vi "Dashboard Main.vi"() -> ()   [LabVIEW 2019]
uses:
  <vilib>/Utility/miscctls.llb/LVRowAndColumnTypeDef.ctl
  <vilib>/event_ctls.llb/eventvkey.ctl
  <vilib>/Rock Robotics/Network Tables/NT Read Numeric Array.vi
  <vilib>/Rock Robotics/WPI/Dashboard/WPI_DashboardLogging Global.vi
  <vilib>/Rock Robotics/Network Tables/NT Read Variant.vi
panel:
  out "NT Connection":bool
  in  "Camera Settings Right":T1={"Frame Rate"=30, "Compression"=30, "Size"=1, "DB Camera Config"=FALSE} {"Frame Rate" scale=1.0..30.0; "Compression" scale=100.0..-1.0; "Size" items=["640x480", "320x240", "160x120"]}
  in  "Camera Name Right":string(combo)="No Camera Selection"
  out "Camera Perf":string
  in  "Camera Settings":T1={"Frame Rate"=30, "Compression"=30, "Size"=1, "DB Camera Config"=FALSE} {"Frame Rate" scale=1.0..30.0; "Compression" scale=100.0..-1.0; "Size" items=["640x480", "320x240", "160x120"]}
  in  "TCP":refnum<k5>
  in  "Rec Mode":enum32{"Stop", "Record", "Playback"}(radio)
  out "Robot IP":string
  out "Image Message":string="Timeout in Camera Communications"
  in  "Dashboard Tab":T2(tab)
  out "SensorData":T3={"LeftDistance"=3962.033502451172, "RightDistance"=3821.920006201172, "LeftVelocity"=0.0, "RightVelocity"=0.0, "Angle"=-59.4, "Location"={597.0445781606653, 278.6835922961287}}
  out "Mode":T4(ring)=enum."Auto Disabled"
  out "Right Camera Perf":cluster{"Bandwidth (Mbps)":dbl, "FPS":dbl}
  out "AutoFilesOnRobot":string[](array[string])
  in  "WaitAtStartOfAuto":dbl
  in  "AutoFileName (No .txt)":string
  out "Camera Image Right":T5(plugin-control)
  in  "DB/String 9":string
  in  "DB/String 8":string
  in  "DB/String 7":string
  in  "DB/String 6":string
  in  "DB/String 5":string
  in  "DB/String 4":string
  in  "DB/String 3":string
  in  "DB/String 2":string
  in  "DB/String 1":string
  in  "DB/String 0":string
  in  "DB/Slider 0":dbl(slide) scale=0.0..5.0
  in  "DB/Slider 1":dbl(slide) scale=0.0..5.0
  in  "DB/Slider 2":dbl(slide) scale=0.0..5.0
  in  "DB/Slider 3":dbl(slide) scale=0.0..5.0
  out "DB/LED 3":bool
  out "DB/LED 2":bool
  out "DB/LED 1":bool
  out "DB/LED 0":bool
  in  "DB/Button 3":bool
  in  "DB/Button 2":bool
  in  "DB/Button 1":bool
  in  "DB/Button 0":bool caption="New Name"
  in  "Test Slider":dbl(slide) scale=0.0..100.0 scale format="%#_3g"
  in  "On/Off":bool caption="Solenoid"
  in  "Test Name":u16(ring) items=["Select the test to run..."]
  in  "Test Tree":string(tree)
  in  "Motor":cluster{"Value":dbl, "Enable":bool} {"Value" scale=-1.0..1.0 scale format="%#_3g"}
  out "Progress":T6 {"Test Progress" scale=0.0..100.0}
  in  "Rev/Fwd":cluster{"Forward":bool, "Reverse":bool}
  in  "Test Ring":u16(ring) items=["Monochrome", "Color"]
  out "Cmd Status":string
  in  "Execute Command":bool
  in  "Command Params":string[][](table)
  in  "Command Selection":i32(listbox)
  in  "CheckList":i32(listbox)
  out "Tree":string(tree)
  out "Camera Image":T5(plugin-control)
  in  "Camera Name":string(combo)="No Camera Selection"
  # "HW"
  # "HW"
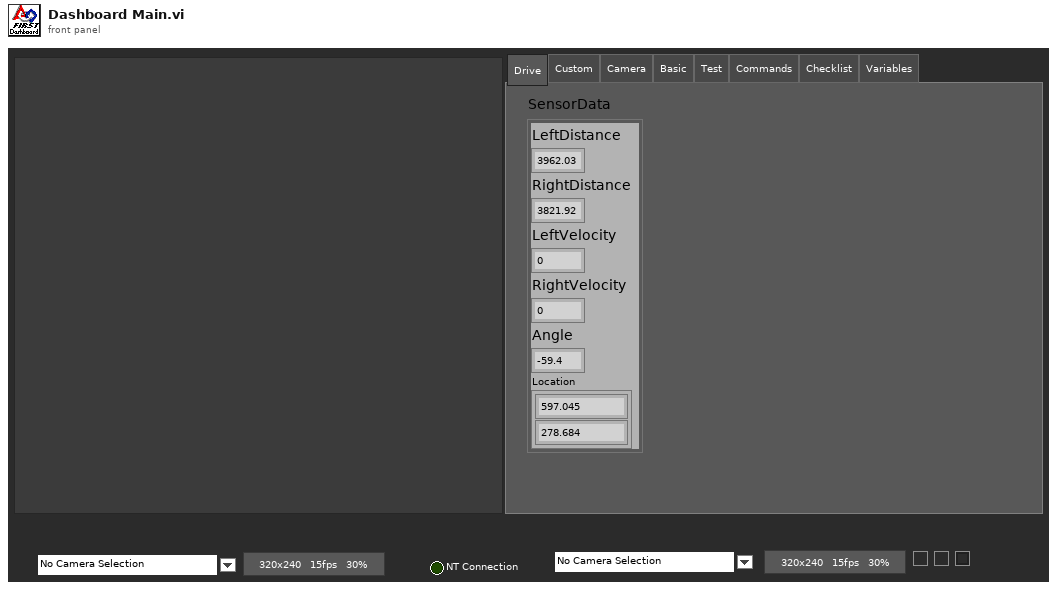
[diagram p1: front panel]
types:
  T1 = cluster{"Frame Rate":i32, "Compression":i32, "Size":u16, "DB Camera Config":bool}
  T2 = enum32{"Drive", "Custom", "Camera", "Basic", "Test", "Commands", "Checklist", "Variables"}
  T3 = cluster{"LeftDistance":dbl, "RightDistance":dbl, "LeftVelocity":dbl, "RightVelocity":dbl, "Angle":dbl, "Location":cluster{dbl, dbl}}
  T4 = enum8{"Tele-Op Disabled", "Tele-Op Enabled", "Auto Disabled", "Auto Enabled", "Test Disabled", "Test Enabled", "Disconnected", "No Code", "E-Stop"}
  T5 = typedef "IMAQ Image.ctl" = refnum<image>
  T6 = cluster{"Test Progress":u8, "Test Progress Text":string}
  T7 = cluster{"Save Path":path, "Interval (s)":dbl, "Keep":i32}
  T8 = typedef "Image Type" = u32
  T9 = cluster{"IDs":cluster{"RPC field ID":u16, "Unique ID":u16}, "String":string}
  T10 = cluster{"Camera Image":refnum<vi>, "Dashboard Tab":refnum<vi>, void, "Rec Mode":refnum<vi>, "Test Slider":refnum<vi>, "On/Off ":refnum<vi>, "Test Ring":refnum<vi>, "Rev/Fwd":refnum<vi>, "Test Name":refnum<vi>, "Motor":refnum<vi>, "Progress":refnum<vi>, "CheckList":refnum<vi>, "Tree":refnum<vi>, "Test Tree":refnum<vi>, "Command Params":refnum<vi>, "Command Selection":refnum<vi>, "Execute Command":refnum<vi>, "Cmd Status":refnum<vi>, "Camera Settings":refnum<vi>, "Camera Name":refnum<vi>, "Camera Perf":refnum<vi>, "Camera Settings Right":refnum<vi>, "Camera Name Right":refnum<vi>, "Camera Image Right":refnum<vi>}
  T11 = cluster{"Error Strings":string, "Disable Counts":cluster{u16, u16}, "Rail Faults":cluster{u16, u16, u16}, "Robot IP":string, "DB Mode":u8, "Event Info":cluster{"Name":string, "Type":u8, "Number":u16, "Replay":u8}}
  T12 = cluster{"Storage":cluster{"Disk Free":u64, "RAM Block":u32, "RAM free":u32}, "CPU Utilization":cluster{"CPU % ISR":sgl, "CPU % Time Crit":sgl, "CPU % Timed Str":sgl, "CPU % High":sgl, "CPU % Above":sgl, "CPU % Normal":sgl, "CPU % Low":sgl}, "CAN":cluster{"% Bus Utilization":sgl, "Bus Off Cnt":u32, "TX_FIFO Full Cnt":u32, "Receive Error Cnt":u8, "Transmit Error Cnt":u8}, "HID":cluster{"HID Outputs":u32, "Rumble Low":u16, "Rumble High":u16}[]}
  T13 = cluster{"Status bits":cluster{"Test Mode":bool, "Autonomous":bool, "Enabled":bool, "Code Start":bool, "Brownout":bool, "Reserved 2":bool, "Reserved 3":bool, "E-Stop":bool}, "Code Trace":cluster{"Disabled":bool, "TeleOp":bool, "Auto":bool, "Test":bool}, "Controller Type":enum16{"unknown", "cRIO", "roboRio"}, "Code?":enum16{"unknown", "noCode", "code"}, "Battery V":dbl}
  T14 = cluster{"Control Bits":cluster{"TestMode":bool, "Autonomous":bool, "Enabled":bool, "FMS Present":bool, bool, bool, bool, "E-Stop":bool}, "Team Station ":u8, "Countdown":sgl, "Joystick Values":cluster{"Axes":dbl[], "Buttons":bool[], "POVs":i16[]}[]}
  T15 = cluster{"Axes":dbl[], "Buttons":bool[], "POVs":i16[]}[]
  T16 = cluster{"Axes":dbl[], "Buttons":bool[], "POVs":i16[]}
  T17 = cluster{"Global Rectangle":i32[], "Contours":cluster{"Contour Type":u32, "ROI Type":u32, "Points":i32[]}[]}
  T18 = cluster{"Camera Name":string, string, "Saved DB Images Info":cluster{"Save Path":path, "Interval (s)":dbl, "Keep":i32}}
  T19 = cluster{"Camera Name Right":string, string, "Saved DB Images Info":cluster{"Save Path":path, "Interval (s)":dbl, "Keep":i32}}
  T20 = cluster{"Operation":enum16{"Update", "Clear"}, "Color Box":u32}[]
  T21 = typedef "eventvkey.ctl" = enum16{"ASCII", "Enter", "Return", "Shift", "Ctrl", "Alt", "Cmd", "Opt", "Caps", "NumLock", "Clear", "Break", "Up", "Down", "Left", "Right", "Insert", "Delete", "Home", "End", "PageUp", "PageDown", "Escape", "Help", "Pause", "ScrollLock", "F1", "F2", "F3", "F4", "F5", "F6", "F7", "F8", "F9", "F10", "F11", "F12", "F13", "F14", "F15", "F16", "F17", "F18", "F19", "F20", "F21", "F22", "F23", "F24", "Play", "VolumeUp", "VolumeDown", "Mute", "Two Byte Char"}
  T22 = cluster{"Image Size":bool, "Image Type":bool, "Pixel Value":bool, "ROI Information":bool, "Zoom Factor":bool}
  T23 = cluster{"Operation":enum16{"Update", "Clear"}, "Color Box":u32}
  T24 = typedef "LVRowAndColumnTypeDef.ctl" = cluster{"Row":i32, "Column":i32}
  T25 = cluster{"Shift":bool, "Ctrl":bool, "Alt":bool, "Cmd":bool, "Opt":bool}
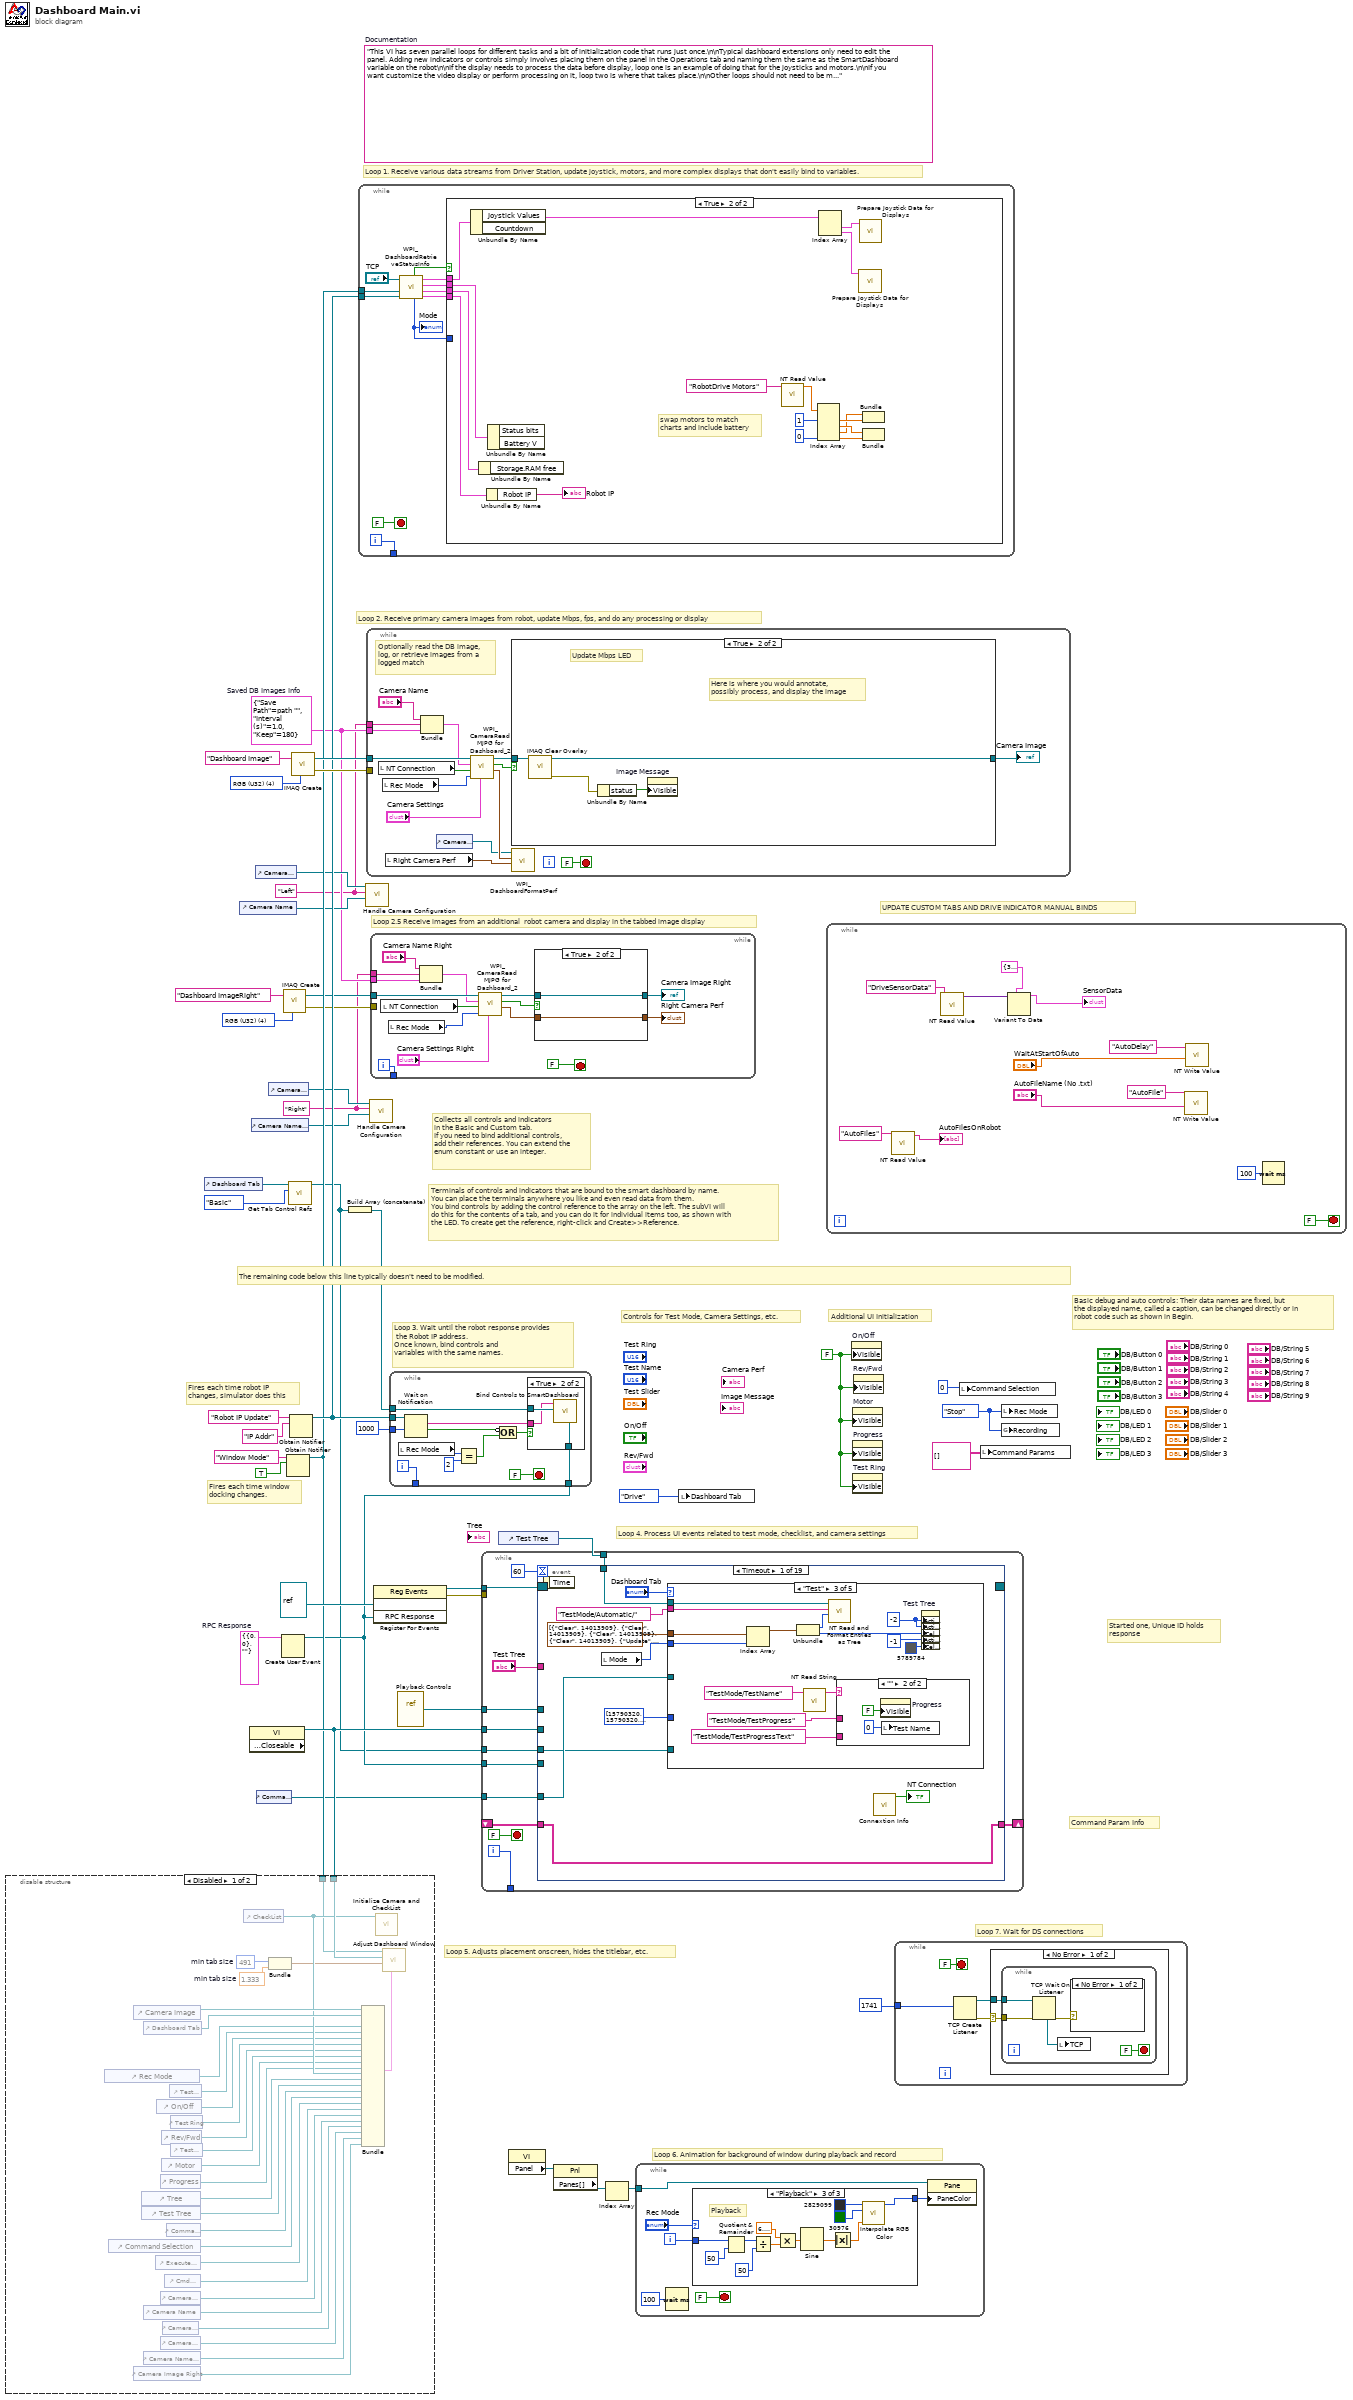
[diagram p0: block diagram]
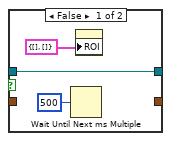
[diagram p3: hidden frame]
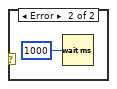
[diagram p4: hidden frame]
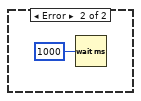
[diagram p5: hidden frame]
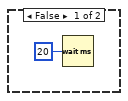
[diagram p6: hidden frame]
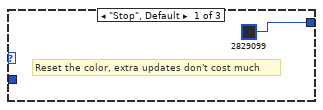
[diagram p7: hidden frame]
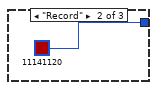
[diagram p8: hidden frame]
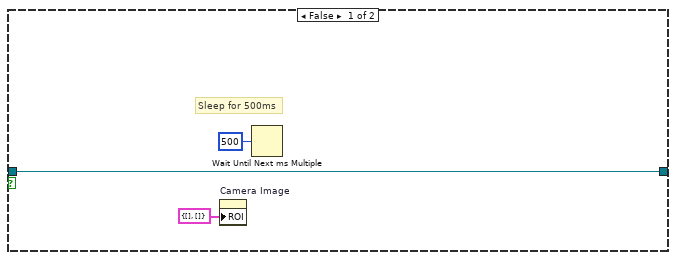
[diagram p10: hidden frame]
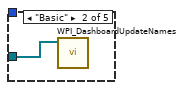
[diagram p12: hidden frame]
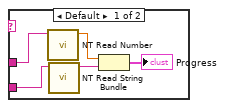
[diagram p13: hidden frame]
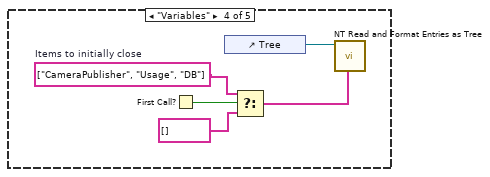
[diagram p14: hidden frame]
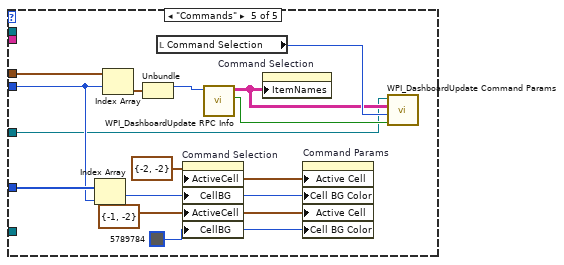
[diagram p15: hidden frame]
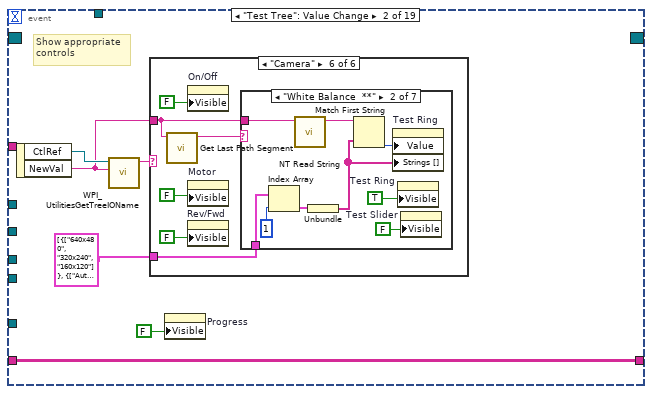
[diagram p16: hidden frame]
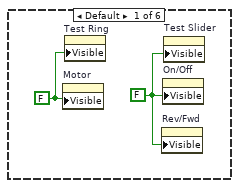
[diagram p17: hidden frame]
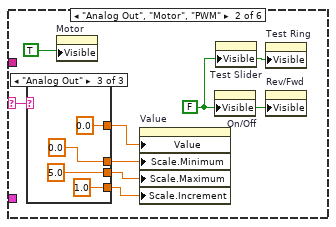
[diagram p18: hidden frame]
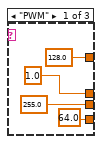
[diagram p19: hidden frame]
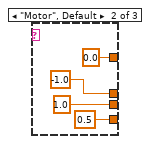
[diagram p20: hidden frame]
diagram:
  w4 = T7 {"Save Path"=path "", "Interval (s)"=1.0, "Keep"=180}  # Saved DB Images Info
  w3 = "Right"
  w2 = "Left"
  w9 = T8 4 items=["Grayscale (U8)", "Grayscale (I16)", "Grayscale (SGL)", "Complex (CSG)", "RGB (U32)", "HSL (U32)", "RGB (U64)"] ("Image Type")
  w18 = T9 {"IDs"={"RPC field ID"=0, "Unique ID"=0}, "String"=""}  # RPC Response
  w27 = enum32{"Stop", "Record", "Playback"}."Stop" ("Rec Mode")
  w23 = FALSE ("Visible")
  (unwired) "This VI has seven parallel loops for different tasks and a bit of initialization code that runs just once.\n\nTypical dashboard extensions only need to edit the panel. Adding new indicators or controls simply involves placing them on the panel in the Operations tab and naming them the same as the SmartDashboard variable on the robot\n\nIf the display needs to process the data before display, loop one is an example of doing that for the joysticks and motors.\n\nIf you want customize the video display or perform processing on it, loop two is where that takes place.\n\nOther loops should not need to be modified. They are pretty standard, and document the task they perform."  # Documentation
  w44 = T8 4 items=["Grayscale (U8)", "Grayscale (I16)", "Grayscale (SGL)", "Complex (CSG)", "RGB (U32)", "HSL (U32)", "RGB (U64)"] ("Image Type")
  # "UPDATE CUSTOM TABS AND DRIVE INDICATOR MANUAL BINDS"
  # "Loop 2.5 Receive images from an additional  robot camera and display in the tabbed image display"
  # "Command Param Info"
  # "Started one, Unique ID holds\nresponse"
  # "Loop 7. Wait for DS connections"
  # "Basic debug and auto controls: Their data names are fixed, but\nthe displayed name, called a caption, can be changed directly or in\nrobot code such as shown in Begin."
  # "Controls for Test Mode, Camera Settings, etc."
  # "Additional UI Initialization"
  # "Loop 6. Animation for background of window during playback and record"
  # "Fires each time robot IP\nchanges, simulator does this"
  # "Fires each time window\ndocking changes."
  # "Collects all controls and indicators\nin the Basic and Custom tab.\nIf you need to bind additional controls,\nadd their references. You can extend the\nenum constant or use an integer."
  # "The remaining code below this line typically doesn't need to be modified."
  # "Loop 4. Process UI events related to test mode, checklist, and camera settings"
  # "Terminals of controls and indicators that are bound to the smart dashboard by name.\nYou can place the terminals anywhere you like and even read data from them.\nYou bind controls by adding the control reference to the array on the left. The subVI will\ndo this for the contents of a tab, and you can do it for individual items too, as shown with\nthe LED. To create get the reference, right-click and Create>>Reference."
  # "Loop 3. Wait until the robot response provides\n the Robot IP address.\nOnce known, bind controls and\nvariables with the same names."
  # "Loop 5. Adjusts placement onscreen, hides the titlebar, etc."
  # "Loop 1. Receive various data streams from Driver Station, update joystick, motors, and more complex displays that don't easily bind to variables."
  # "Loop 2. Receive primary camera images from robot, update Mbps, fps, and do any processing or display"
  n1 = control-ref of="Dashboard Tab"() -> (w25:refnum<vi>)
  n2 = control-ref of="Camera Name"() -> (w12:refnum<vi>)
  n3 = property class="VI" props=["Front Panel.Closeable"]() -> (reference out=w26:refnum<vi>)  [unwired: 2 in, 2 out]
  n4 = control-ref of="Camera Name Right"() -> (w5:refnum<vi>)
  n5 = control-ref of="Camera Settings"() -> (w13:refnum<vi>)
  n6 = control-ref of="Command Params"() -> (w14:refnum<vi>)
  n7 = control-ref of="Camera Settings Right"() -> (w6:refnum<vi>)
  n8 = Create User Event(user event datatype=w18) -> (user event=w15:refnum<user-event>)  [unwired: 1 in, 1 out]
  n9 = call "IMAQ Create"("Image Name"="Dashboard ImageRight", "Image Type"=w9) -> ("New Image"=w8:T5, "error out"=w7:errorcluster)  [unwired: 2 in, 1 out]
  n10 = Obtain Notifier(name (unnamed)="Window Mode", notification data type=TRUE) -> (notifier out=w21:refnum<notifier>)  [unwired: 2 in, 2 out]
  n11 = disable-structure shown="Disabled" {
    disable-tunnel: w26 -> [w73 _]
    disable-tunnel: w21 -> [w58 _]
    frame Disabled {
      w47 = 491  # min tab size
      w46 = 1.333  # min tab size
      n12 = control-ref of="Rec Mode"() -> (w64:refnum<vi>)
      n13 = control-ref of="Command Selection"() -> (w55:refnum<vi>)
      n14 = control-ref of="Camera Image Right"() -> (w48:refnum<vi>)
      n15 = control-ref of="Camera Image"() -> (w72:refnum<vi>)
      n16 = control-ref of="Tree"() -> (w68:refnum<vi>)
      n17 = control-ref of="Test Tree"() -> (w67:refnum<vi>)
      n18 = control-ref of="Dashboard Tab"() -> (w71:refnum<vi>)
      n19 = control-ref of="Camera Name"() -> (w52:refnum<vi>)
      n20 = control-ref of="Camera Name Right"() -> (w49:refnum<vi>)
      n21 = control-ref of="Execute Command"() -> (w56:refnum<vi>)
      n22 = control-ref of="On/Off"() -> (w62:refnum<vi>)
      n23 = control-ref of="Progress"() -> (w59:refnum<vi>)
      n24 = control-ref of="Camera Settings"() -> (w53:refnum<vi>)
      n25 = control-ref of="Camera Settings Right"() -> (w50:refnum<vi>)
      n26 = control-ref of="Rev/Fwd"() -> (w60:refnum<vi>)
      n27 = control-ref of="Motor"() -> (w65:refnum<vi>)
      n28 = control-ref of="Camera Perf"() -> (w51:refnum<vi>)
      n29 = control-ref of="Cmd Status"() -> (w54:refnum<vi>)
      n30 = control-ref of="Command Params"() -> (w57:refnum<vi>)
      n31 = control-ref of="Test Slider"() -> (w63:refnum<vi>)
      n32 = control-ref of="Test Ring"() -> (w61:refnum<vi>)
      n33 = control-ref of="Test Name"() -> (w66:refnum<vi>)
      n34 = control-ref of="CheckList"() -> (w69:refnum<vi>)
      n35 = Bundle("min tab size"=w47, "min tab size"=w46) -> (w45:cluster{"min tab size":i32, "min tab size":dbl})  [unwired: 1 in]
      n36 = Bundle("Camera Image"=w72, "Dashboard Tab"=w71, "Rec Mode"=w64, "Test Slider"=w63, "On/Off"=w62, "Test Ring"=w61, "Rev/Fwd"=w60, "Test Name"=w66, "Motor"=w65, "Progress"=w59, "CheckList"=w69, "Tree"=w68, "Test Tree"=w67, "Command Params"=w57, "Command Selection"=w55, "Execute Command"=w56, "Cmd Status"=w54, "Camera Settings"=w53, "Camera Name"=w52, "Camera Perf"=w51, "Camera Settings Right"=w50, "Camera Name Right"=w49, "Camera Image Right"=w48) -> (w70:T10)  [unwired: 2 in]
      n37 = call "Initialize Camera and CheckList.vi"("ListBox in"=w69) -> ()  [unwired: 11 in]
      n38 = call "Adjust Dashboard Window.vi"("Sizing Refnums"=w70, "Size Constraints"=w45, "VI"=w73, "WIn Mode"=w58) -> ()  [unwired: 8 in]
    }
    frame Enabled {
    }
  }
  n39 = call <vilib>:"Get Tab Control Refs.vi"("Page Index"=T2."Basic" ("Dashboard Tab"), "TabControl in"=w25) -> ("ControlsOnPage"=w11:refnum<vi>[])  [unwired: 9 in]
  n40 = Obtain Notifier(name (unnamed)="Robot IP Update", notification data type="IP Addr" ("name (unnamed)")) -> (notifier out=w22:refnum<notifier>)  [unwired: 2 in, 2 out]
  n41 = call "IMAQ Create"("Image Name"="Dashboard Image", "Image Type"=w44) -> ("New Image"=w42:T5, "error out"=w41:errorcluster)  [unwired: 2 in, 1 out]
  n42 = Build Array (concatenate)(w11) -> (w24:refnum<vi>[])
  n43 = while {
    tunnel: [w83] -> _
    tunnel: w22 -> [w77]
    tunnel: w21 -> [w74]
    i -> [w83]
    stop <- FALSE stop-if-true
    n44 = call <vilib>:"WPI_DashboardRetrieveStatusInfo.vi"("Binding Refnum"=w77, "Window Mode Notifier"=w74, "TCP Cnx"="TCP") -> ("Power and Errors"=w78:T11, "Robot Metrics"=w81:T12, "Status Info"=w82:T13, "Control Info"=w79:T14, "Robot Mode"=w76:T4, "Process?"=w80:bool)  [unwired: 3 in]
    "Mode" <- w76
    n45 = case shown="True" w80 {
      tunnel: w82 -> [_ w101]
      tunnel: w81 -> [_ w100]
      tunnel: w79 -> [_ w99]
      tunnel: w78 -> [_ w98]
      tunnel: w76 -> [_ _]
      frame False {
        n46 = Wait (ms)(milliseconds to wait=u32 20) -> ()  [unwired: 1 out]
      }
      frame True {
        # "swap motors to match\ncharts and include battery"
        n47 = Unbundle By Name(w99) -> ("Joystick Values"=w91:T15)  [unwired: 1 out]
        n48 = Unbundle By Name(w100) -> ()  [unwired: 1 out]
        n49 = Unbundle By Name(w98) -> ("Robot IP"=→"Robot IP":string)
        n50 = Unbundle By Name(w101) -> ()  [unwired: 2 out]
        n51 = call-poly <vilib>:"NT Read Value.vi"("Name"="RobotDrive Motors") -> ("Numeric Array"=w87:dbl[])  [unwired: 9 in, 1 out]
        n52 = Index Array(array=w87, index #1=1, index #4=0) -> (element #1=w93:dbl, element #2=w94:dbl, element #3=w92:dbl, element #4=w97:dbl)  [unwired: 2 in]
        n53 = Index Array(array=w91) -> (element #1=w90:T16, element #2=w89:T16)  [unwired: 2 in]
        n54 = call "Prepare Joystick Data for Displays.vi"("Joystick Values"=w89) -> ()  [unwired: 8 in, 3 out]
        n55 = call "Prepare Joystick Data for Displays.vi"("Joystick Values"=w90) -> ()  [unwired: 8 in, 3 out]
        n56 = Bundle("Numeric"=w92, "Numeric"=w93) -> ()  [unwired: 1 in, 1 out]
        n57 = Bundle("Numeric"=w94, "Numeric"=w97) -> ()  [unwired: 1 in, 1 out]
      }
    }
  }
  n58 = call "Handle Camera Configuration.vi"("CameraNameRef"=w12, "Display Name"=w2, "ClusterRef"=w13) -> ()  [unwired: 9 in]
  n59 = while {
    tunnel: w42 -> [w115]
    tunnel: w41 -> [_]
    tunnel: w4 -> [w108]
    tunnel: w2 -> [w105]
    stop <- FALSE stop-if-true
    # "Optionally read the DB image,\nlog, or retrieve images from a\nlogged match"
    n60 = local read "NT Connection"() -> (w109:bool)
    n61 = local read "Rec Mode"() -> (w112:enum32{"Stop", "Record", "Playback"})
    n62 = local read "Right Camera Perf"() -> (w103:cluster{"Bandwidth (Mbps)":dbl, "FPS":dbl})
    n63 = Bundle("Camera Name"="Camera Name", w105, "Saved DB Images Info"=w108) -> (w107:T18)  [unwired: 1 in]
    n64 = control-ref of="Camera Perf"() -> (w102:refnum<vi>)
    n65 = call <vilib>:"WPI_CameraRead MJPG for Dashboard_2.vi"("Camera Settings"="Camera Settings", "Rec Mode"=w112, "NT Connection"=w109, "Capture Info"=w107, "Image in"=w115) -> ("perf info"=w104:cluster{"Bandwidth (Mbps)":dbl, "fps":dbl}, "Active"=w113:bool, "Image\\ out"=w114:T5)  [unwired: 4 in]
    n66 = case shown="True" w113 {
      tunnel: w114 -> [w118 w121]
      tunnel: [w118 w120] -> w110
      frame False {
        # "Sleep for 500ms"
        n67 = property on="Camera Image" class="ImageControl"("ROI"=T17 {"Global Rectangle"=[], "Contours"=[]}) -> ()  [unwired: 2 in, 2 out]
        n68 = Wait Until Next ms Multiple(millisecond multiple=u32 500) -> ()  [unwired: 1 out]
      }
      frame True {
        # "Here is where you would annotate,\npossibly process, and display the image"
        # "Update Mbps LED"
        n69 = call "IMAQ Clear Overlay"("Image"=w121) -> ("error out"=w122:errorcluster, "Image Out"=w120:T5)  [unwired: 2 in, 7 out]
        n70 = Unbundle By Name(w122) -> ("status"=w123:bool)
        n71 = property on="Image Message" class="Str"("Visible"=w123) -> ()  [unwired: 2 in, 2 out]
      }
    }
    "Camera Image" <- w110
    n72 = call <vilib>:"WPI_DashboardFormatPerf.vi"("Right Camera Perf"=w103, "Performance"=w104, "String in"=w102) -> ()  [unwired: 9 in]
  }
  n73 = call "Handle Camera Configuration.vi"("CameraNameRef"=w5, "Display Name"=w3, "ClusterRef"=w6) -> ()  [unwired: 9 in]
  n74 = while {
    tunnel: w8 -> [w138]
    tunnel: w7 -> [_]
    tunnel: [w133] -> _
    tunnel: w4 -> [w129]
    tunnel: w3 -> [w126]
    i -> [w133]
    stop <- FALSE stop-if-true
    n75 = local read "NT Connection"() -> (w130:bool)
    n76 = local read "Rec Mode"() -> (w137:enum32{"Stop", "Record", "Playback"})
    n77 = Bundle("Camera Name Right"="Camera Name Right", w126, "Saved DB Images Info"=w129) -> (w128:T19)  [unwired: 1 in]
    n78 = call <vilib>:"WPI_CameraRead MJPG for Dashboard_2.vi"("Camera Settings"="Camera Settings Right", "Rec Mode"=w137, "NT Connection"=w130, "Capture Info"=w128, "Image in"=w138) -> ("perf info"=w124:cluster{"Bandwidth (Mbps)":dbl, "fps":dbl}, "Active"=w132:bool, "Image\\ out"=w135:T5)  [unwired: 4 in]
    n79 = case shown="True" w132 {
      tunnel: w135 -> [w140 w143]
      tunnel: [w140 w143] -> w131
      tunnel: [_ w142] -> w125
      tunnel: w124 -> [_ w142]
      frame False {
        n80 = Wait Until Next ms Multiple(millisecond multiple=u32 500) -> ()  [unwired: 1 out]
        n81 = property on="Camera Image Right" class="ImageControl"("ROI"=T17 {"Global Rectangle"=[], "Contours"=[]}) -> ()  [unwired: 2 in, 2 out]
      }
      frame True {
      }
    }
    "Camera Image Right" <- w131
    "Right Camera Perf" <- w125
  }
  n82 = register-events(refnum<vi> refnum, w15) -> (reference out=w31:refnum<event-registration>, error out=w30:errorcluster)  [unwired: 2 in]
  n83 = while {
    tunnel: w24 -> [w155]
    tunnel: w22 -> [w153]
    tunnel: [w151] -> _
    tunnel: u32 1000 ("milliseconds to wait") -> [w150]
    tunnel: w15 -> [w144]
    i -> [w151]
    stop <- FALSE stop-if-true
    n84 = local read "Rec Mode"() -> (w146:enum32{"Stop", "Record", "Playback"})
    n85 = Wait on Notification(notifier=w153, timeout in ms (-1)=w150) -> (notification=w152:string, timed out?=w148:bool)  [unwired: 2 in, 2 out]
    n86 = Equal?(x=w146, y=u16 2 ("Rec Mode")) -> (x = y?=w147:bool)
    n87 = Compound Arithmetic op=OR(invert w148, w147) -> (w149:bool)
    n88 = case shown="True" w149 {
      tunnel: w155 -> [_ w158]
      tunnel: w152 -> [_ w157]
      tunnel: w144 -> [_ w156]
      frame False {
      }
      frame True {
        n89 = call <vilib>:"Bind Controls to SmartDashboard.vi"("RPC ref"=w156, "Bound Control Refs"=w158, "Server IP Address"=w157) -> ()  [unwired: 9 in]
      }
    }
  }
  n90 = vi-ref "Playback Controls.vi"() -> (w32:refnum<vi>)
  n91 = control-ref of="Test Tree"() -> (w36:refnum<vi>)
  n92 = while {
    tunnel: [w168] -> _
    tunnel: w36 -> [w167]
    tunnel: w32 -> [w166]
    tunnel: w31 -> [w165]
    tunnel: w30 -> [_]
    tunnel: w26 -> [w164]
    tunnel: w15 -> [w163]
    tunnel: w14 -> [w162]
    shift-right: [w161] -> _
    shift-left: _ -> [w160]
    tunnel: w11 -> [w159]
    i -> [w168]
    stop <- FALSE stop-if-true
    n93 = event shown="[0] Timeout" {
      selector: w165 -> [_ _ _ _ _ _ _ _ _ _ _ _ _ _ _ _ _ _ _]
      dyn-events: [_ _ _ _ _ _ _ _ _ _ _ _ _ _ w422 _ _ _ _] -> _
      timeout: u32 60 ("milliseconds to wait") -> [_ _ _ _ _ _ _ _ _ _ _ _ _ _ _ _ _ _ _]
      tunnel: w167 -> [w180 _ _ _ _ _ _ _ _ _ _ _ _ _ _ _ _ _ _]
      tunnel: "Test Tree" -> [_ _ _ _ _ _ _ _ _ w389 w397 w399 w403 w411 _ _ _ _ _]
      tunnel: w166 -> [_ _ _ _ _ _ _ _ _ _ _ _ _ _ w424 _ w442 _ _]
      tunnel: w164 -> [_ _ _ _ _ _ _ _ _ _ _ _ _ _ w420 _ _ _ _]
      tunnel: w163 -> [_ _ _ _ _ _ _ _ _ _ _ _ _ _ w418 _ _ _ _]
      tunnel: w162 -> [w175 _ _ _ w340 _ _ _ _ _ _ _ _ _ _ _ _ _ _]
      tunnel: [w174 w223 w325 w330 w338 w347 w357 w364 w376 w388 w395 w398 w402 w410 w417 w437 w439 w443 w456] -> w161
      tunnel: w160 -> [w174 w223 w325 w330 w338 _ _ w364 w376 w388 w395 w398 w402 w410 w417 w437 w439 w443 w456]
      tunnel: w159 -> [w172 _ _ _ _ _ _ _ _ _ _ _ _ _ _ _ _ _ _]
      event Timeout {
        n94 = event-data() -> ()  [unwired: 1 in, 1 out]
        n95 = local read "Mode"() -> (w177:T4)
        n96 = case shown="\"Test\"" "Dashboard Tab" {
          tunnel: w180 -> [_ _ w196 _ _]
          tunnel: "TestMode/Automatic/" ("Name Pattern") -> [_ _ w195 _ _]
          tunnel: T20 [{"Operation"=enum."Clear", "Color Box"=14013909}, {"Operation"=enum."Clear", "Color Box"=14013909}, {"Operation"=enum."Clear", "Color Box"=14013909}, {"Operation"=enum."Clear", "Color Box"=14013909}, {"Operation"=enum."Update", "Color Box"=14013909}, {"Operation"=enum."Update", "Color Box"=16777215}, {"Operation"=enum."Clear", "Color Box"=14013909}, {"Operation"=enum."Clear", "Color Box"=14013909}, {"Operation"=enum."Clear", "Color Box"=14013909}] -> [_ _ w188 _ w216]
          tunnel: w177 -> [_ _ w187 _ w215]
          tunnel: u32[] [15790320, 15790320, 15790320, 15790320, 16777215, 16777215, 15790320, 15790320, 15790320] -> [_ _ _ _ w221]
          tunnel: w175 -> [_ _ _ _ w209]
          tunnel: w172 -> [_ w182 _ _ _]
          frame "Custom", Default {
          }
          frame "Basic" {
            n97 = call <vilib>:"WPI_DashboardUpdateNames.vi"("Controls on Tab"=w182) -> ()  [unwired: 11 in]
          }
          frame "Test" {
            w194 = -2 ("Active Item:Row Number")
            n98 = Index Array(array=w188, index=w187) -> (element=w189:T23)
            n99 = Unbundle(w189) -> ("Operation"=w190:enum16{"Update", "Clear"}, "Color Box"=w191:u32)
            n100 = call <vilib>:"NT Read String.vi"("Name"="TestMode/TestName") -> ("String"=w185:string)  [unwired: 9 in, 1 out]
            n101 = call <vilib>:"NT Read and Format Entries as Tree.vi"("Operation"=w190, "Name Pattern"=w195, "Tree Refnum"=w196) -> ()  [unwired: 7 in, 2 out]
            n102 = case shown="\"\"" w185 {
              tunnel: "TestMode/TestProgress" ("Name") -> [w198 _]
              tunnel: "TestMode/TestProgressText" ("Name") -> [w197 _]
              frame Default {
                n103 = call <vilib>:"NT Read Number.vi"("Name"=w198) -> ("Numeric"=w199:dbl)  [unwired: 9 in, 1 out]
                n104 = call <vilib>:"NT Read String.vi"("Name"=w197) -> ("String"=w200:string)  [unwired: 9 in, 1 out]
                n105 = Bundle("Numeric"=w199, "String"=w200) -> (→"Progress":cluster{"Numeric":dbl, "String":string})  [unwired: 1 in]
              }
              frame "" {
                n106 = property on="Progress" class="Clust (strict)"("Visible"=FALSE) -> ()  [unwired: 2 in, 2 out]
                n107 = local write "Test Name"(u16 0) -> ()
              }
            }
            n108 = property on="Test Tree" class="Tree (strict)"("Active Item Row Number"=w194, "ActiveColNum"=w194, "CellBG"=w191, "Active Item Row Number"=-1 ("Active Item:Row Number"), "CellBG"=u32 5789784 ("Color Box")) -> ()  [unwired: 2 in, 2 out]
          }
          frame "Variables" {
            w206 = string[] ["CameraPublisher", "Usage", "DB"]  # Items to initially close
            n109 = First Call?() -> (First Call?: T/F=w207:bool)
            n110 = control-ref of="Tree"() -> (w208:refnum<vi>)
            n111 = Select(t=w206, s=w207, f=string[] []) -> (s? t:f=w204:string[])
            n112 = call <vilib>:"NT Read and Format Entries as Tree.vi"("Tags to  Close"=w204, "Tree Refnum"=w208) -> ()  [unwired: 8 in, 2 out]
          }
          frame "Commands" {
            w217 = u32 5789784 ("Color Box")
            w218 = T24 {"Row"=-1, "Column"=-2} ("Active Cell:Active Cell")
            w220 = T24 {"Row"=-2, "Column"=-2} ("Active Cell:Active Cell")
            n113 = Index Array(array=w221, index=w215) -> (element=w219:u32)
            n114 = Index Array(array=w216, index=w215) -> (element=w214:T23)
            n115 = Unbundle(w214) -> ("Operation"=w213:enum16{"Update", "Clear"})  [unwired: 1 out]
            n116 = local read "Command Selection"() -> (w212:i32)
            n117 = property on="Command Selection" class="MCListbox (strict)"("ActiveCell"=w220, "CellBG"=w219, "ActiveCell"=w218, "CellBG"=w217) -> ()  [unwired: 2 in, 2 out]
            n118 = call <vilib>:"WPI_DashboardUpdate RPC Info.vi"("Operation"=w213) -> ("update"=w211:bool, "commands"=w210:string[][])  [unwired: 9 in]
            n119 = property on="Command Selection" class="MCListbox (strict)"("ItemNames"=w210) -> ()  [unwired: 2 in, 2 out]
            n120 = property on="Command Params" class="Tbl (strict)"("Active Cell"=w220, "Cell BG Color"=w219, "Active Cell"=w218, "Cell BG Color"=w217) -> ()  [unwired: 2 in, 2 out]
            n121 = call <vilib>:"WPI_DashboardUpdate Command Params.vi"("Update"=w211, "NewVal"=w212, "Commands"=w210, "Param Tbl"=w209) -> ()  [unwired: 7 in, 1 out]
          }
        }
        n122 = call <vilib>:"Connextion Info.vi"() -> ("Connected"=→"NT Connection":bool)  [unwired: 10 in, 1 out]
      }
      event "Test Tree": Value Change {
        # "Show appropriate\ncontrols"
        n123 = event-data() -> ("CtlRef"=w226:refnum<vi>, "NewVal"=w224:string)  [unwired: 1 in]
        n124 = call <vilib>:"WPI_UtilitiesGetTreeIOName.vi"("NewVal"=w224, "TreeControl in"=w226) -> ("I/O Name"=w227:string)  [unwired: 9 in]
        n125 = case shown="\"Camera\"" w227 {
          selector: w227 -> [_ w234 _ w256 w265 _]
          tunnel: w224 -> [_ _ w253 w255 _ w272]
          tunnel: cluster{string[]}[] [{["640x480", "320x240", "160x120"]}, {["Auto", "Fixed indoor", "Fixed outdoor 1", "Fixed outdoor 2", "Fixed fluorescent 1", "Fixed fluorescent 2", "Hold current"]}, {["Auto", "Flicker-free 50 Hz", "Flicker-free 60 Hz", "Hold current"]}, {["None", "Prioritize frame rate", "Prioritize image quality"]}, {["Monochrome", "Color"]}] -> [_ _ _ _ _ w271]
          frame Default {
            w229 = FALSE ("Visible")
            w228 = FALSE ("Visible")
            n126 = property on="Motor" class="Clust (strict)"("Visible"=w228) -> ()  [unwired: 2 in, 2 out]
            n127 = property on="Test Ring" class="Ring (strict)"("Visible"=w228) -> ()  [unwired: 2 in, 2 out]
            n128 = property on="Rev/Fwd" class="Clust (strict)"("Visible"=w229) -> ()  [unwired: 2 in, 2 out]
            n129 = property on="On/Off" class="Bool (strict)"("Visible"=w229) -> ()  [unwired: 2 in, 2 out]
            n130 = property on="Test Slider" class="Slide (strict)"("Visible"=w229) -> ()  [unwired: 2 in, 2 out]
          }
          frame "Analog Out", "Motor", "PWM" {
            w235 = FALSE ("Visible")
            n131 = case shown="\"Analog Out\"" w234 {
              tunnel: [1.0 ("Value") -1.0 ("Value") 0.0 ("Value")] -> w233
              tunnel: [255.0 ("Value") 1.0 ("Value") 5.0 ("Value")] -> w232
              tunnel: [128.0 ("Value") 0.0 ("Value") 0.0 ("Value")] -> w231
              tunnel: [64.0 ("Value") 0.5 ("Value") 1.0 ("Value")] -> w230
              frame "PWM" {
              }
              frame "Motor", Default {
              }
              frame "Analog Out" {
              }
            }
            n132 = property on="Motor" class="Clust (strict)"("Visible"=TRUE) -> ()  [unwired: 2 in, 2 out]
            n133 = property on="Value" class="Slide (strict)"("Value"=w231, "Scale.Minimum"=w233, "Scale.Maximum"=w232, "Scale.Increment"=w230) -> ()  [unwired: 2 in, 2 out]
            n134 = property on="On/Off" class="Bool (strict)"("Visible"=w235) -> ()  [unwired: 2 in, 2 out]
            n135 = property on="Test Slider" class="Slide (strict)"("Visible"=w235) -> ()  [unwired: 2 in, 2 out]
            n136 = property on="Test Ring" class="Ring (strict)"("Visible"=w235) -> ()  [unwired: 2 in, 2 out]
            n137 = property on="Rev/Fwd" class="Clust (strict)"("Visible"=w235) -> ()  [unwired: 2 in, 2 out]
          }
          frame "Servo" {
            w251 = FALSE ("Visible")
            n138 = call <vilib>:"NT Read Number.vi"("Name"=w253) -> ("Numeric"=w252:dbl)  [unwired: 9 in, 1 out]
            n139 = property on="Test Slider" class="Slide (strict)"("Visible"=TRUE, "Scale.Maximum"=170.0 ("Scale.Range:Maximum")) -> ()  [unwired: 2 in, 2 out]
            n140 = local write "Test Slider"(w252) -> ()
            n141 = property on="Motor" class="Clust (strict)"("Visible"=w251) -> ()  [unwired: 2 in, 2 out]
            n142 = property on="Rev/Fwd" class="Clust (strict)"("Visible"=w251) -> ()  [unwired: 2 in, 2 out]
            n143 = property on="On/Off" class="Bool (strict)"("Visible"=w251) -> ()  [unwired: 2 in, 2 out]
            n144 = property on="Test Ring" class="Ring (strict)"("Visible"=w251) -> ()  [unwired: 2 in, 2 out]
          }
          frame "Relay", "Solenoid" {
            w254 = FALSE ("Visible")
            n145 = property on="Motor" class="Clust (strict)"("Visible"=w254) -> ()  [unwired: 2 in, 2 out]
            n146 = property on="Test Slider" class="Slide (strict)"("Visible"=w254) -> ()  [unwired: 2 in, 2 out]
            n147 = Search and Replace String(input string=w255, search string="/Value  **", replace string="/Direction") -> (result string=w261:string)  [unwired: 5 in, 3 out]
            n148 = property on="Test Ring" class="Ring (strict)"("Visible"=w254) -> ()  [unwired: 2 in, 2 out]
            n149 = call <vilib>:"NT Read String.vi"("Name"=w261) -> ("String"=w259:string)  [unwired: 9 in, 1 out]
            n150 = Equal?(x="Both directions", y=w259) -> (x = y?=w257:bool)
            n151 = Not(x=w257) -> (.not. x?=w258:bool)
            n152 = property on="Rev/Fwd" class="Clust (strict)"("Visible"=w257) -> ()  [unwired: 2 in, 2 out]
            n153 = property on="On/Off" class="Bool (strict)"("Visible"=w258, "Caption.Text"=w256) -> ()  [unwired: 2 in, 2 out]
          }
          frame "Compressor", "Digital Out" {
            w264 = FALSE ("Visible")
            # "Get direction and finish"
            n154 = property on="Motor" class="Clust (strict)"("Visible"=w264) -> ()  [unwired: 2 in, 2 out]
            n155 = property on="Test Slider" class="Slide (strict)"("Visible"=w264) -> ()  [unwired: 2 in, 2 out]
            n156 = property on="Test Ring" class="Ring (strict)"("Visible"=w264) -> ()  [unwired: 2 in, 2 out]
            n157 = property on="On/Off" class="Bool (strict)"("Visible"=TRUE, "Caption.Text"=w265) -> ()  [unwired: 2 in, 2 out]
            n158 = property on="Rev/Fwd" class="Clust (strict)"("Visible"=FALSE) -> ()  [unwired: 2 in, 2 out]
          }
          frame "Camera" {
            n159 = call <vilib>:"Get Last Path Segment.vi"("String in"=w272) -> ("String out"=w273:string)  [unwired: 10 in]
            n160 = property on="On/Off" class="Bool (strict)"("Visible"=FALSE) -> ()  [unwired: 2 in, 2 out]
            n161 = property on="Motor" class="Clust (strict)"("Visible"=FALSE) -> ()  [unwired: 2 in, 2 out]
            n162 = property on="Rev/Fwd" class="Clust (strict)"("Visible"=FALSE) -> ()  [unwired: 2 in, 2 out]
            n163 = case shown="\"White Balance  **\"" w273 {
              tunnel: w272 -> [w279 w288 w297 w306 w315 _ w321]
              tunnel: w271 -> [w277 w285 w294 w303 w312 _ _]
              frame "Size  **" {
                n164 = Index Array(array=w277) -> (element=w276:cluster{string[]})  [unwired: 1 in]
                n165 = call <vilib>:"NT Read String.vi"("Name"=w279) -> ("String"=w278:string)  [unwired: 9 in, 1 out]
                n166 = Unbundle(w276) -> (w274:string[])
                n167 = Match First String(2:w274, 3:w278) -> (0:w275:i32)  [unwired: 1 out]
                n168 = property on="Test Ring" class="Ring (strict)"("Value"=w275, "Strings []"=w274) -> ()  [unwired: 2 in, 2 out]
                n169 = property on="Test Ring" class="Ring (strict)"("Visible"=TRUE) -> ()  [unwired: 2 in, 2 out]
                n170 = property on="Test Slider" class="Slide (strict)"("Visible"=FALSE) -> ()  [unwired: 2 in, 2 out]
              }
              frame "White Balance  **" {
                n171 = Index Array(array=w285, index=1) -> (element=w286:cluster{string[]})
                n172 = call <vilib>:"NT Read String.vi"("Name"=w288) -> ("String"=w287:string)  [unwired: 9 in, 1 out]
                n173 = Unbundle(w286) -> (w283:string[])
                n174 = Match First String(2:w283, 3:w287) -> (0:w282:i32)  [unwired: 1 out]
                n175 = property on="Test Ring" class="Ring (strict)"("Value"=w282, "Strings []"=w283) -> ()  [unwired: 2 in, 2 out]
                n176 = property on="Test Ring" class="Ring (strict)"("Visible"=TRUE) -> ()  [unwired: 2 in, 2 out]
                n177 = property on="Test Slider" class="Slide (strict)"("Visible"=FALSE) -> ()  [unwired: 2 in, 2 out]
              }
              frame "Exposure  **" {
                n178 = Index Array(array=w294, index=2) -> (element=w295:cluster{string[]})
                n179 = call <vilib>:"NT Read String.vi"("Name"=w297) -> ("String"=w296:string)  [unwired: 9 in, 1 out]
                n180 = Unbundle(w295) -> (w291:string[])
                n181 = Match First String(2:w291, 3:w296) -> (0:w292:i32)  [unwired: 1 out]
                n182 = property on="Test Ring" class="Ring (strict)"("Value"=w292, "Strings []"=w291) -> ()  [unwired: 2 in, 2 out]
                n183 = property on="Test Ring" class="Ring (strict)"("Visible"=TRUE) -> ()  [unwired: 2 in, 2 out]
                n184 = property on="Test Slider" class="Slide (strict)"("Visible"=FALSE) -> ()  [unwired: 2 in, 2 out]
              }
              frame "Exposure Priority  **" {
                n185 = Index Array(array=w303, index=3) -> (element=w304:cluster{string[]})
                n186 = call <vilib>:"NT Read String.vi"("Name"=w306) -> ("String"=w305:string)  [unwired: 9 in, 1 out]
                n187 = Unbundle(w304) -> (w300:string[])
                n188 = Match First String(2:w300, 3:w305) -> (0:w301:i32)  [unwired: 1 out]
                n189 = property on="Test Ring" class="Ring (strict)"("Value"=w301, "Strings []"=w300) -> ()  [unwired: 2 in, 2 out]
                n190 = property on="Test Ring" class="Ring (strict)"("Visible"=TRUE) -> ()  [unwired: 2 in, 2 out]
                n191 = property on="Test Slider" class="Slide (strict)"("Visible"=FALSE) -> ()  [unwired: 2 in, 2 out]
              }
              frame "Color Enable  **" {
                n192 = Index Array(array=w312, index=4) -> (element=w313:cluster{string[]})
                n193 = call <vilib>:"NT Read String.vi"("Name"=w315) -> ("String"=w314:string)  [unwired: 9 in, 1 out]
                n194 = Unbundle(w313) -> (w309:string[])
                n195 = Match First String(2:w309, 3:w314) -> (0:w310:i32)  [unwired: 1 out]
                n196 = property on="Test Ring" class="Ring (strict)"("Value"=w310, "Strings []"=w309) -> ()  [unwired: 2 in, 2 out]
                n197 = property on="Test Ring" class="Ring (strict)"("Visible"=TRUE) -> ()  [unwired: 2 in, 2 out]
                n198 = property on="Test Slider" class="Slide (strict)"("Visible"=FALSE) -> ()  [unwired: 2 in, 2 out]
              }
              frame Default {
                n199 = property on="Test Ring" class="Ring (strict)"("Visible"=FALSE) -> ()  [unwired: 2 in, 2 out]
                n200 = property on="Test Slider" class="Slide (strict)"("Visible"=FALSE) -> ()  [unwired: 2 in, 2 out]
              }
              frame "Brightness  **", "Color Level  **", "Compression  **", "FPS  **", "Sharpness  **" {
                n201 = call <vilib>:"NT Read Number.vi"("Name"=w321) -> ("Numeric"=w320:dbl)  [unwired: 9 in, 1 out]
                n202 = local write "Test Slider"(w320) -> ()
                n203 = property on="Test Slider" class="Slide (strict)"("Visible"=TRUE, "Scale.Maximum"=100.0 ("Scale.Range:Maximum")) -> ()  [unwired: 2 in, 2 out]
                n204 = property on="Test Ring" class="Ring (strict)"("Visible"=FALSE) -> ()  [unwired: 2 in, 2 out]
              }
            }
          }
        }
        n205 = property on="Progress" class="Clust (strict)"("Visible"=FALSE) -> ()  [unwired: 2 in, 2 out]
      }
      event "Test Name": Mouse Enter {
        # "Populate the ring with the list of tests"
        n206 = event-data() -> ()  [unwired: 1 in, 1 out]
        n207 = call <vilib>:"NT Read String Array.vi"("Name"="TestMode/TestList") -> ("String Array"=w329:string[])  [unwired: 9 in, 1 out]
        n208 = Build Array (concatenate)("Select the test to run...", w329) -> (w328:string[])
        n209 = property on="Test Name" class="Ring (strict)"("Strings []"=w328) -> ()  [unwired: 2 in, 2 out]
      }
      event "Test Name": Value Change {
        w331 = FALSE ("Visible")
        # "Tell the robot the test name to run"
        n210 = event-data() -> ("NewVal"=w335:u16)  [unwired: 1 in]
        n211 = property on="Test Name" class="Ring (strict)"() -> ("Strings []"=w336:string[])  [unwired: 2 in, 2 out]
        n212 = local write "Progress"(T6 {"Test Progress"=0, "Test Progress Text"=""} ("Progress")) -> ()
        n213 = Index Array(array=w336, index=w335) -> (element=w334:string)
        n214 = call <vilib>:"NT Write String.vi"("String"=w334, "Name"="TestMode/TestName") -> ()  [unwired: 9 in, 1 out]
        n215 = property on="Progress" class="Clust (strict)"("Visible"=TRUE) -> ()  [unwired: 2 in, 2 out]
        n216 = property on="Motor" class="Clust (strict)"("Visible"=w331) -> ()  [unwired: 2 in, 2 out]
        n217 = property on="Test Slider" class="Slide (strict)"("Visible"=w331) -> ()  [unwired: 2 in, 2 out]
        n218 = property on="On/Off" class="Bool (strict)"("Visible"=w331) -> ()  [unwired: 2 in, 2 out]
        n219 = property on="Rev/Fwd" class="Clust (strict)"("Visible"=w331) -> ()  [unwired: 2 in, 2 out]
        n220 = property on="Test Ring" class="Ring (strict)"("Visible"=w331) -> ()  [unwired: 2 in, 2 out]
      }
      event "Command Selection": Value Change {
        # "Get the params and show in table"
        n221 = event-data() -> ("NewVal"=w341:i32)  [unwired: 1 in]
        n222 = property on="Command Selection" class="MCListbox (strict)"() -> ("ItemNames"=w339:string[][])  [unwired: 2 in, 2 out]
        n223 = call <vilib>:"WPI_DashboardUpdate Command Params.vi"("NewVal"=w341, "Commands"=w339, "Param Tbl"=w340) -> ()  [unwired: 8 in, 1 out]
      }
      event "Execute Command": Value Change {
        # "Started one, Unique ID holds\nresponse"
        n224 = event-data() -> ()  [unwired: 1 in, 1 out]
        n225 = property on="Command Selection" class="MCListbox (strict)"() -> ("ItemNames"=w352:string[][])  [unwired: 2 in, 2 out]
        n226 = Index Array(array=w352, index (row)="Command Selection", index (col)=0) -> (element=w350:string)
        n227 = call <vilib>:"Invoke Commands.vi"("Command Params"="Command Params", "Function Name"=w350) -> ("Params"=w346:u8, "Started"=w345:bool)  [unwired: 7 in, 1 out]
        n228 = Array Subset(array="Command Params", length (row)=w346) -> (w347:string[][])  [unwired: 3 in]
        n229 = Select(t="Executing" ("Cmd Status"), s=w345, f="" ("Cmd Status")) -> (s? t:f=→"Cmd Status":string)
      }
      event "Command Selection": Double Click {
        n230 = event-data() -> ("Row"=w360:i32)  [unwired: 1 in]
        n231 = property on="Command Selection" class="MCListbox (strict)"() -> ("ItemNames"=w363:string[][])  [unwired: 2 in, 2 out]
        n232 = local read "Command Params"() -> (w359:string[][])
        n233 = Index Array(array=w363, index (row)=w360, index (col)=0) -> (element=w361:string)
        n234 = call <vilib>:"Invoke Commands.vi"("Command Params"=w359, "Function Name"=w361) -> ("Params"=w358:u8, "Started"=w353:bool)  [unwired: 7 in, 1 out]
        n235 = Array Subset(array=w359, length (row)=w358) -> (w357:string[][])  [unwired: 3 in]
        n236 = Select(t="Executing" ("Cmd Status"), s=w353, f="" ("Cmd Status")) -> (s? t:f=w354:string)
        n237 = local write "Cmd Status"(w354) -> ()
      }
      event "CheckList": Double Click {
        # "Shift clears all"
        # "Update symbols on the listbox"
        n238 = event-data() -> ("PlatMods.Shift"=w365:bool, "Row"=w367:i32)  [unwired: 1 in]
        n239 = case shown="True" w365 {
          tunnel: w367 -> [w371 _]
          tunnel: 1 -> [w370 _]
          frame False {
            n240 = property on="CheckList" class="LstBox (strict)"() -> ("Item Symbols"=w369:i32[])  [unwired: 2 in, 2 out]
            n241 = Replace Array Subset(array=w369, new element=w370, index=w371) -> (w368:i32[])
            n242 = property on="CheckList" class="LstBox (strict)"("Item Symbols"=w368) -> ()  [unwired: 2 in, 2 out]
          }
          frame True {
            w372 = 0 ("Top Row")
            n243 = property on="CheckList" class="LstBox (strict)"() -> ("Number of Rows"=w374:u32)  [unwired: 2 in, 2 out]
            n244 = Initialize Array(0, w374) -> (w373:i32[])
            n245 = property on="CheckList" class="LstBox (strict)"("Top Row"=w372, "Value"=w372, "Item Symbols"=w373) -> ()  [unwired: 2 in, 2 out]
          }
        }
      }
      event "CheckList": Key Down {
        # "Update symbols on the listbox\nLeft and right keys check and uncheck"
        n246 = event-data() -> ("VKey"=w378:T21)  [unwired: 1 in]
        n247 = case shown="\"Left\", \"Right\"" w378 {
          selector: w378 -> [w383 _]
          tunnel: eventvkey."Left" ("VKey") -> [w381 _]
          frame "Left", "Right" {
            n248 = Equal?(x=w381, y=w383) -> (x = y?=w382:bool)
            n249 = Select(t=0, s=w382, f=1) -> (s? t:f=w384:i32)
            n250 = property on="CheckList" class="LstBox (strict)"() -> ("Item Symbols"=w387:i32[])  [unwired: 2 in, 2 out]
            n251 = Replace Array Subset(array=w387, new element=w384, index="CheckList") -> (w386:i32[])
            n252 = property on="CheckList" class="LstBox (strict)"("Item Symbols"=w386) -> ()  [unwired: 2 in, 2 out]
          }
          frame Default {
          }
        }
      }
      event "Motor.Enable": Value Change {
        # "When the test mode otor enable helper is set, update that\ntree row item's value"
        n253 = event-data() -> ("NewVal"=w393:bool)  [unwired: 1 in]
        n254 = Unbundle("Motor") -> ("Value"=w392:dbl)  [unwired: 1 out]
        n255 = Select(t=w392, s=w393, f=0.0) -> (s? t:f=w390:dbl)
        n256 = call <vilib>:"NT Write Number.vi"("Numeric"=w390, "Name"=w389) -> ()  [unwired: 9 in, 1 out]
      }
      event "Test Slider": Value Change {
        # "When the test mode slider helper is set, update that\ntree row item's value"
        n257 = event-data() -> ("NewVal"=w396:dbl)  [unwired: 1 in]
        n258 = call <vilib>:"NT Write Number.vi"("Numeric"=w396, "Name"=w397) -> ()  [unwired: 9 in, 1 out]
      }
      event "On/Off": Value Change {
        # "When the test mode on/off helper value is set, update that\ntree row item's value"
        n259 = event-data() -> ("NewVal"=w401:bool)  [unwired: 1 in]
        n260 = Boolean To (0,1)(Boolean=w401) -> (0, 1=w400:i16)
        n261 = call <vilib>:"NT Write Number.vi"("Numeric"=w400, "Name"=w399) -> ()  [unwired: 9 in, 1 out]
      }
      event "Rev/Fwd": Value Change {
        # "When the test mode helper value for relays is set, update that\ntree row item's value"
        n262 = event-data() -> ("NewVal.Forward"=w409:bool, "NewVal.Reverse"=w408:bool)  [unwired: 1 in]
        n263 = Boolean To (0,1)(Boolean=w409) -> (0, 1=w405:i16)
        n264 = Boolean To (0,1)(Boolean=w408) -> (0, 1=w407:i16)
        n265 = Negate(x=w407) -> (-x=w406:i16)
        n266 = Add(x=w405, y=w406) -> (x+y=w404:i16)
        n267 = call <vilib>:"NT Write Number.vi"("Numeric"=w404, "Name"=w403) -> ()  [unwired: 9 in, 1 out]
      }
      event "Test Ring": Value Change {
        # "When a test mode helper value is selected from the ring,\nset the tree item's variable to the string value"
        n268 = event-data() -> ("NewVal"=w413:u16)  [unwired: 1 in]
        n269 = property on="Test Ring" class="Ring (strict)"() -> ("Strings []"=w414:string[])  [unwired: 2 in, 2 out]
        n270 = Index Array(array=w414, index=w413) -> (element=w412:string)
        n271 = call <vilib>:"NT Write String.vi"("String"=w412, "Name"=w411) -> ()  [unwired: 9 in, 1 out]
      }
      event "Rec Mode": Value Change {
        # "Update globals for recording mode and path to read log from.\nClear when logging and let NetworkTables set path for vision to\nuse."
        n272 = event-data() -> ("NewVal"=w425:enum32{"Stop", "Record", "Playback"})  [unwired: 1 in]
        n273 = global write "WPI_DashboardLogging Global.vi" "Logging Filename"(path "") -> ()
        n274 = global write "WPI_DashboardLogging Global.vi" "Recording"(w425) -> ()
        n275 = case shown="\"Playback\"" w425 {
          tunnel: w424 -> [_ w427 w436]
          tunnel: [_ _ w435] -> w422
          tunnel: [_ _ w434] -> _
          tunnel: w420 -> [_ _ w432]
          tunnel: cluster{i32, i32} {-250, 170} -> [_ _ w431]
          tunnel: [_ _ T22 {"Image Size"=TRUE, "Image Type"=TRUE, "Pixel Value"=TRUE, "ROI Information"=TRUE, "Zoom Factor"=FALSE} ("Image Information Shown:All Elements")] -> w415
          tunnel: [_ _ TRUE ("Zoom Factor")] -> w416
          tunnel: w418 -> [_ _ w428]
          frame Default {
          }
          frame "Stop", "Record" {
            # "Place Window too"
            n276 = invoke class="VI" method="FP.Close"(reference=w427) -> (reference out=w426:refnum<vi>)  [unwired: 2 in, 2 out]
            n277 = invoke class="VI" method="Abort VI"(reference=w426) -> ()  [unwired: 2 in, 3 out]
          }
          frame "Playback" {
            n278 = call "Open Playback Panel.vi"("Offset"=w431, "DB VI Ref"=w432, "Playback in"=w436) -> ("Playback out"=w433:refnum<vi>)  [unwired: 8 in]
            n279 = register-events(w433, w428) -> (reference out=w435:refnum<event-registration>, error out=w434:errorcluster)  [unwired: 2 in]
          }
        }
        n280 = property on="Camera Image Right" class="ImageControl"("Image Information Shown"=w415, "Image Information Visible"=w416) -> ()  [unwired: 2 in, 2 out]
        n281 = property on="Camera Image" class="ImageControl"("Image Information Shown"=w415, "Image Information Visible"=w416) -> ()  [unwired: 2 in, 2 out]
        n282 = call <vilib>:"WPI_DashboardNT Log FieldName Cache.vi"("Operation"=enum16{"Lookup/Add", "Index", "Clear"}."Clear") -> ()  [unwired: 8 in, 3 out]
      }
      event Panel Close {
        w438 = enum32{"Stop", "Record", "Playback"}."Stop" ("Rec Mode")
        # "Playback window has been closed, abort"
        n283 = event-data() -> ()  [unwired: 1 in, 4 out]
        n284 = local write "Rec Mode"(w438) -> ()
        n285 = global write "WPI_DashboardLogging Global.vi" "Recording"(w438) -> ()
      }
      event Panel Close {
        # "Abort playback window and ourself"
        n286 = event-data() -> ()  [unwired: 1 in, 4 out]
        n287 = invoke class="VI" method="FP.Close"(reference=w442) -> (reference out=w441:refnum<vi>)  [unwired: 2 in, 2 out]
        n288 = invoke class="VI" method="Abort VI"(reference=w441) -> (error out=w440:errorcluster)  [unwired: 2 in, 2 out]
        n289 = invoke class="VI" method="Abort VI"(error in=w440) -> ()  [unwired: 2 in, 3 out]
      }
      event User Event {
        n290 = event-data() -> ("IDs"=w449:cluster{"RPC field ID":u16, "Unique ID":u16}, "String"=w448:string)  [unwired: 1 in]
        n291 = Bundle("IDs"=w449, "String"=w448) -> (w447:T9)  [unwired: 1 in]
        n292 = call <vilib>:"Retrieve RPC Response.vi"("RPC Response"=w447) -> ("Output"=w445:string[][])  [unwired: 10 in]
        n293 = Build Array (concatenate)(w443, w445) -> (w444:string[][])
        n294 = local write "Command Params"(w444) -> ()
        n295 = local write "Cmd Status"("" ("Cmd Status")) -> ()
      }
      event "Tree": Double Click {
        n296 = event-data() -> ("PlatMods"=w455:T25, "Tag"=w452:string)  [unwired: 1 in]
        n297 = Unbundle(w455) -> ("Shift"=w454:bool)  [unwired: 4 out]
        n298 = String Subset(string=w452, length (rest)=1 ("length (rest)")) -> (substring=w451:string)  [unwired: 1 in]
        n299 = Not(x=w454) -> (.not. x?=w453:bool)
        n300 = case shown="\"/\"" w451 {
          tunnel: w452 -> [_ w458]
          tunnel: w453 -> [_ w457]
          frame Default {
          }
          frame "/" {
            n301 = call <vilib>:"NT Update Persistence.vi"("Persistence"=w457, "Name"=w458) -> ()  [unwired: 9 in, 1 out]
          }
        }
      }
    }
  }
  n302 = property class="VI"() -> ("Panel"=w34:refnum<vi>)  [unwired: 2 in, 2 out]
  n303 = property class="Pnl"(reference=w34) -> ("Panes[]"=w35:refnum<vi>[])  [unwired: 1 in, 2 out]
  n304 = Index Array(array=w35) -> (element=w33:refnum<vi>)  [unwired: 1 in]
  n305 = while {
    tunnel: w33 -> [w460]
    i -> [w463]
    stop <- FALSE stop-if-true
    n306 = Wait (ms)(milliseconds to wait=u32 100) -> ()  [unwired: 1 out]
    n307 = case shown="\"Playback\"" "Rec Mode" {
      tunnel: w463 -> [_ _ w478]
      tunnel: [u32 2829099 ("Base Color") u32 11141120 ("Target Color") w467] -> w459
      frame "Stop", Default {
        # "Reset the color, extra updates don't cost much"
      }
      frame "Record" {
      }
      frame "Playback" {
        # "Playback"
        n308 = Quotient & Remainder(x=w478, y=u32 50 ("milliseconds to wait")) -> (x-y*floor(x/y)=w474:u32)  [unwired: 1 out]
        n309 = Divide(x=w474, y=u32 50 ("milliseconds to wait")) -> (x/y=w471:dbl)
        n310 = Multiply(x=6.283185307179586, y=w471) -> (x*y=w476:dbl)
        n311 = Sine(x=w476) -> (sin(x)=w475:dbl)
        n312 = Absolute Value(x=w475) -> (abs(x)=w468:dbl)
        n313 = call "Interpolate RGB Color.vi"("Proportion"=w468, "Target Color"=u32 30976, "Base Color"=u32 2829099) -> ("Result Color"=w467:u32)  [unwired: 8 in]
      }
    }
    n314 = property class="Pane"(reference=w460, "PaneColor"=w459) -> ()  [unwired: 1 in, 2 out]
  }
  n315 = local write "Dashboard Tab"(T2."Drive" ("Dashboard Tab")) -> ()
  n316 = while {
    stop <- FALSE stop-if-true
    n317 = call-poly <vilib>:"NT Read Value.vi"("Name"="AutoFiles") -> ("String Array"=→"AutoFilesOnRobot":string[])  [unwired: 9 in, 1 out]
    n318 = call-poly <vilib>:"NT Read Value.vi"("Name"="DriveSensorData") -> ("Variant"=w488:variant)  [unwired: 9 in, 1 out]
    n319 = Variant To Data(type=T3 {"LeftDistance"=3962.033502451172, "RightDistance"=3821.920006201172, "LeftVelocity"=0.0, "RightVelocity"=0.0, "Angle"=-59.4, "Location"={597.0445781606653, 278.6835922961287}} ("SensorData"), Variant=w488) -> (data=→"SensorData":T3)  [unwired: 1 in, 1 out]
    n320 = call-poly <vilib>:"NT Write Value.vi"("String"="AutoFileName (No .txt)", "Name"="AutoFile") -> ()  [unwired: 9 in, 1 out]
    n321 = call-poly <vilib>:"NT Write Value.vi"("Numeric"="WaitAtStartOfAuto", "Name"="AutoDelay") -> ()  [unwired: 9 in, 1 out]
    n322 = Wait (ms)(milliseconds to wait=u32 100) -> ()  [unwired: 1 out]
  }
  n323 = property on="On/Off" class="Bool (strict)"("Visible"=w23) -> ()  [unwired: 2 in, 2 out]
  n324 = property on="Motor" class="Clust (strict)"("Visible"=w23) -> ()  [unwired: 2 in, 2 out]
  n325 = property on="Progress" class="Clust (strict)"("Visible"=w23) -> ()  [unwired: 2 in, 2 out]
  n326 = property on="Test Ring" class="Ring (strict)"("Visible"=w23) -> ()  [unwired: 2 in, 2 out]
  n327 = property on="Rev/Fwd" class="Clust (strict)"("Visible"=w23) -> ()  [unwired: 2 in, 2 out]
  n328 = while {
    tunnel: u16 1741 ("timeout ms (25000)") -> [w492]
    stop <- FALSE stop-if-true
    n329 = TCP Create Listener(10:w492) -> (0:w491:errorcluster, 3:w493:refnum<k5>)  [unwired: 4 in, 1 out]
    n330 = case shown="No Error" w491 {
      selector: w491 -> [w495 _]
      tunnel: w493 -> [w496 _]
      frame No Error {
        n331 = while {
          tunnel: w496 -> [w499]
          tunnel: w495 -> [w498]
          stop <- FALSE stop-if-true
          n332 = TCP Wait On Listener(8:w498, 11:w499) -> (0:w500:errorcluster, 4:w501:refnum<k5>)  [unwired: 2 in, 3 out]
          n333 = local write "TCP"(w501) -> ()
          n334 = case shown="No Error" w500 {
            frame No Error {
            }
            frame Error {
              n335 = Wait (ms)(milliseconds to wait=u32 1000) -> ()  [unwired: 1 out]
            }
          }
        }
      }
      frame Error {
        n336 = Wait (ms)(milliseconds to wait=u32 1000) -> ()  [unwired: 1 out]
      }
    }
  }
  n337 = local write "Command Selection"(u16 0 ("milliseconds to wait")) -> ()
  n338 = local write "Command Params"(string[][] [] ("Command Params")) -> ()
  n339 = global write "WPI_DashboardLogging Global.vi" "Recording"(w27) -> ()
  n340 = local write "Rec Mode"(w27) -> ()
